vi "Stop Triggers.vi"(8 "Error in":errorcluster, 10 "Alazar Task":refnum<k21>, 11 "AFG11000 Task":refnum<k21>) -> (0 "error out":errorcluster)   [LabVIEW 2014]
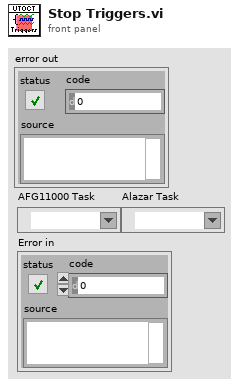
[diagram p1: front panel]
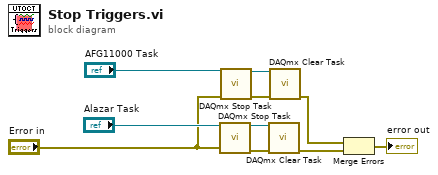
[diagram p0: block diagram]
diagram:
  n1 = call <vilib>:"DAQmx Stop Task.vi"("task/channels in"="Alazar Task", "error in"="Error in") -> ("task out"=w9:refnum<k21>, "error out"=w8:errorcluster)  [unwired: 12 in]
  n2 = call <vilib>:"DAQmx Stop Task.vi"("task/channels in"="AFG11000 Task", "error in"="Error in") -> ("task out"=w6:refnum<k21>, "error out"=w7:errorcluster)  [unwired: 12 in]
  n3 = call <vilib>:"DAQmx Clear Task.vi"("task in"=w9, "error in"=w8) -> ("error out"=w3:errorcluster)  [unwired: 13 in]
  n4 = call <vilib>:"DAQmx Clear Task.vi"("task in"=w6, "error in"=w7) -> ("error out"=w2:errorcluster)  [unwired: 13 in]
  n5 = Merge Errors(w2, w3) -> (→"error out":errorcluster)
